vi "ExCascadeCircBufROI.vi"() -> ()   [LabVIEW 2010]
panel:
  in  "ADC Gain":u32
  out "ADC Speed (Khz)":u32
  in  "Fast ADC":bool
  in  "Avalanche Gain\nOnly valid for \nport 0":dbl format="%.2f"
  in  "OverLap Mode":bool
  in  "ReadOut Port":u32 max=1 step=1
  in  "X Start":u32=1 min=1 step=1
  in  "Y Bin":u32=1 min=1 step=1
  in  "X End":u32=512 min=1 max=512 step=1
  in  "X Bin":u32=1 min=1 step=1
  in  "Y Start":u32=1 min=1 step=1
  in  "Y End":u32=512 min=1 max=512 step=1
  in  "Temperature":dbl=-10.0 format="%.2f"
  in  "Exposure":dbl min=0.0 step=0.001 format="%.3f"
  in  "stop":bool
  in  "Store":bool
  out "error out":errorcluster
  in  "error in (no error)":errorcluster
  # "ExCascadeCircBufROI:\nThis example allows a single ROI\nto be programmed up. It then runs\nin sync (focus) mode displaying \nthe ROI data as it comes in.\nNote: this example requires the \ncamera support circular buffers.\nThis example also shows how to \nsetup the cascade to run in over-\nlapped mode and how to set the\non-chip multiplication gain and how\nto set the readout port."
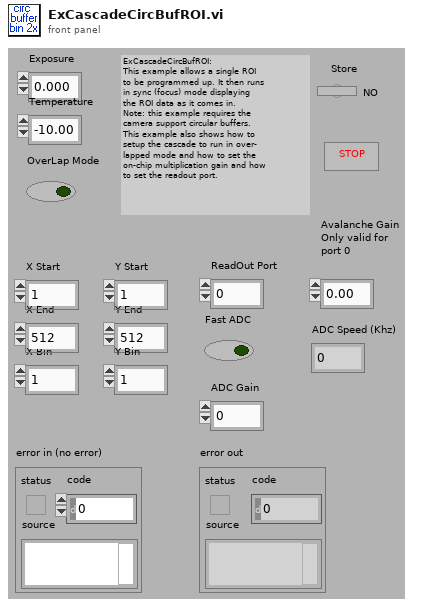
[diagram p1: front panel]
types:
  T1 = cluster{"X Start":u32, "X End":u32, "X Bin":u32, "Y Start":u32, "Y End":u32, "Y Bin":u32}
  T2 = cluster{"acquire focus mode":u32, "Exposure":dbl, "Number of Images":u32, "Software accumulation":u32}
  T3 = cluster{"Camera Handle":u32, "Pulser Handle":u32, "File Handle":u32, "Display Handle":u32, "Image Handle":u32}
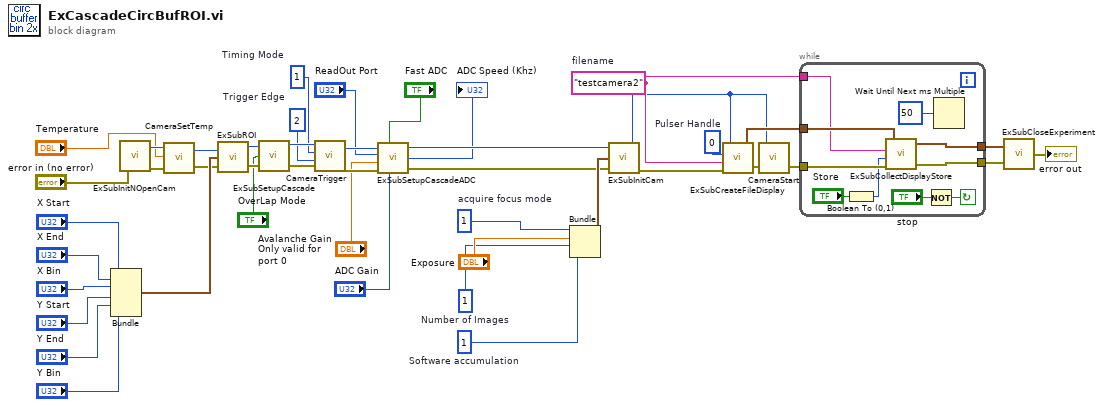
[diagram p0: block diagram]
diagram:
  w27 = u32 0  # Pulser Handle
  w28 = u32 1  # Timing Mode
  w29 = u32 2  # Trigger Edge
  w32 = u32 1  # acquire focus mode
  w31 = u32 1  # Number of Images
  w30 = u32 1  # Software accumulation
  w44 = "testcamera2"  # filename
  n1 = Bundle("X Start"="X Start", "X End"="X End", "X Bin"="X Bin", "Y Start"="Y Start", "Y End"="Y End", "Y Bin"="Y Bin") -> (w19:T1)  [unwired: 1 in]
  n2 = call "ExSubInitNOpenCam.vi"("error in (no error)"="error in (no error)") -> ("Camera Handle"=w16:u32, "error out"=w17:errorcluster)
  n3 = call <userlib>:"CameraSetTemp.vi"("error in (no error)"=w17, "Temperature"="Temperature", "Camera Handle"=w16) -> ("error out"=w15:errorcluster, "Camera Handle"=w14:u32)
  n4 = call "ExSubROI.vi"("error in (no error)"=w15, "ROI"=w19, "Camera Handle"=w14) -> ("error out"=w12:errorcluster, "Camera Handle"=w18:u32)
  n5 = call "ExSubSetupCascade.vi"("error in (no error)"=w12, "OverLap Mode"="OverLap Mode", "Camera Handle"=w18) -> ("error out"=w11:errorcluster, "Camera Handle"=w35:u32)
  n6 = call <userlib>:"CameraTrigger.vi"("error in"=w11, "Trigger Edge"=w29, "Timing Mode"=w28, "Camera Handle"=w35) -> ("error out"=w8:errorcluster, "Camera Handle"=w9:u32)
  n7 = call "ExSubSetupCascadeADC.vi"("Camera Handle"=w9, "Fast ADC"="Fast ADC", "ReadOut Port"="ReadOut Port", "Avalanche Gain\nOnly valid for \nport 0"="Avalanche Gain\nOnly valid for \nport 0", "ADC Gain"="ADC Gain", "error in (no error)"=w8) -> ("Camera Handle"=w6:u32, "ADC Speed (Khz)"=→"ADC Speed (Khz)":u32, "error out"=w7:errorcluster)
  n8 = Bundle("acquire focus mode"=w32, "Exposure"="Exposure", "Number of Images"=w31, "Software accumulation"=w30) -> (w41:T2)  [unwired: 1 in]
  n9 = call "ExSubInitCam.vi"("error in (no error)"=w7, "Camera Information"=w41, "Camera Handle"=w6) -> ("error out"=w40:errorcluster, "Camera Handle"=w26:u32)
  n10 = call "ExSubCreateFileDisplay.vi"("error in (no error)"=w40, "File and Display Name"=w44, "Pulser Handle"=w27, "Camera Handle"=w26) -> ("error out"=w33:errorcluster, "Handles Out"=w39:T3)
  n11 = call <userlib>:"CameraStart.vi"("error in"=w33, "Camera Handle"=w26) -> ("error out"=w34:errorcluster)  [unwired: 1 out]
  n12 = while {
    tunnel: w39 -> [w53]
    tunnel: w34 -> [w52]
    tunnel: w44 -> [w45]
    tunnel: [w50] -> w37
    tunnel: [w51] -> w38
    stop <- w48 continue-if-true
    n13 = Boolean To (0,1)(Boolean="Store") -> (0, 1=w46:i16)
    n14 = call "ExSubCollectDisplayStore.vi"("error in (no error)"=w52, "Store flag"=w46, "Display Title"=w45, "Handle Cluster"=w53) -> ("error out"=w50:errorcluster, "Handle Cluster Out"=w51:T3)  [unwired: 1 out]
    n15 = Not(x="stop") -> (.not. x?=w48:bool)
    n16 = Wait Until Next ms Multiple(millisecond multiple=u32 50) -> ()  [unwired: 1 out]
  }
  n17 = call "ExSubCloseExperiment.vi"("error in (no error)"=w37, "Handles In"=w38) -> ("error out"=→"error out":errorcluster)
